vi "PT100Circuit.vi"(11 "temp":dbl) -> (3 "voltage":dbl)   [LabVIEW 2020]
doc: "Simulates the conversion of temperature to voltage as performed by a PT100 with its conditioning circuit."
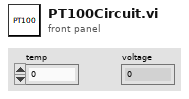
[diagram p1: front panel]
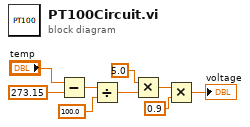
[diagram p0: block diagram]
diagram:
  n1 = Subtract(x="temp", y=273.15) -> (x-y=w3:dbl)
  n2 = Divide(x=w3, y=100.0) -> (x/y=w5:dbl)
  n3 = Multiply(x=5.0, y=w5) -> (x*y=w7:dbl)
  n4 = Multiply(x=w7, y=0.9) -> (x*y=→"voltage":dbl)
